vi "stack_Omega.vi"(2 "error in (no error)":errorcluster, 3 "\\phi(t)":T1, 4 "Omega":T1) -> (0 "error out":errorcluster, 1 "New Omega":T1)   [LabVIEW 2021]
uses:
  <vilib>/Analysis/Matrix/Datatypes/RealMatrix.ctl
  <vilib>/Analysis/Matrix/NI_Matrix.lvlib
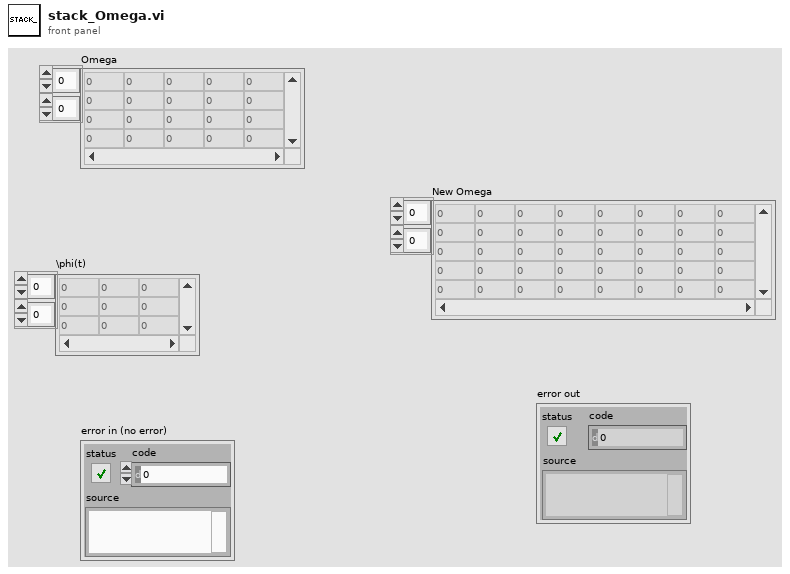
[diagram p1: front panel]
types:
  T1 = typedef "NI_Matrix.lvlib/RealMatrix.ctl" = dbl[][]
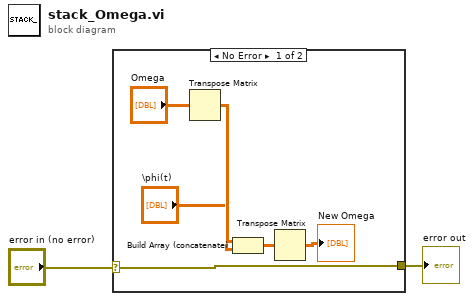
[diagram p0: block diagram]
diagram:
  n1 = case shown="No Error" "error in (no error)" {
    selector: "error in (no error)" -> [w4 w9]
    tunnel: [w4 w9] -> w1
    frame No Error {
      n2 = Transpose Matrix(1:"Omega") -> (0:w7:T1)
      n3 = Build Array (concatenate)(w7, "\\phi(t)") -> (w6:T1)
      n4 = Transpose Matrix(1:w6) -> (0:→"New Omega":T1)
    }
    frame Error {
    }
  }
  "error out" <- w1
